vi "Inline HW RT Driver VI.vi"(7 "Operation":T1, 11 "Device Reference in":T2 format="%.0x") -> (0 "Error Code":i32)   [LabVIEW 2023, in "Waveform Analog Output Engine.lvlib"]
uses:
  Waveform Analog Output Engine.lvlib
  <vilib>/NI VeriStand/Custom Device API/Custom Device Item Ref.ctl
  <vilib>/NI VeriStand/Custom Device API/Hardware Interface Driver VI Operation.ctl
  <vilib>/NI VeriStand/Custom Device API/Custom Device Channel Type.ctl
  <vilib>/NI VeriStand/Custom Device API/Data Access Type.ctl
  <vilib>/NI VeriStand/Custom Device API/Block Data Reference.ctl
  <vilib>/NI VeriStand/Custom Device API/Data Reference.ctl
  DAQ Config Data.ctl
  Shared/Constants.vi
  <vilib>/NI VeriStand/Custom Device API/Global Data Refs.vi
  <vilib>/NI VeriStand/Custom Device API/Custom Device API.lvlib
  <resource>/objmgr/daqmx.rc
  Shared/Waveform Analog Output Shared.lvlib
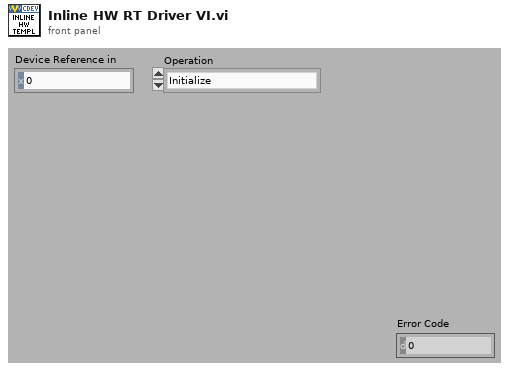
[diagram p1: front panel]
types:
  T1 = typedef "Custom Device API.lvlib/Hardware Interface Driver VI Operation.ctl" = enum16{"Initialize", "Start", "Read Data from HW", "Write Data to HW", "Close"}
  T2 = typedef "Custom Device API.lvlib/Custom Device Item Ref.ctl" = u64
  T3 = typedef "Custom Device API.lvlib/Block Data Reference.ctl" = cluster{"Data Reference":T4, "Offset":u64, "Length":u64}
  T4 = typedef "Custom Device API.lvlib/Data Reference.ctl" = i32
  T5 = typedef "Waveform Analog Output Engine.lvlib/DAQ Config Data.ctl" = cluster{"DAQ Physical Channel(s)":string, "SampleRate":dbl, "MaxV":dbl, "MinV":dbl, "#Samples":dbl, "StartDelay(ms)":dbl, "#OutputBuffers":dbl, "# Channels":i32, "Actual Sample Rate":dbl, "DAQ Ref Out":refnum<k21>, "Latency":dbl}
  T6 = cluster{"Input Data Refs":T3[], "Input Values Array":dbl[], "Output Data Refs":T3[], "Output Values Array":dbl[], "System Config Data":T5, "Error":errorcluster, "Waveform Parameter FIFO":refnum<k33>}
  T7 = cluster{"read mode":enum16{"polling", "blocking"}, "write mode":enum16{"polling", "blocking"}}
  T8 = cluster{"Hw Max":dbl, "Hw Min":dbl, "Requested Amplitude":dbl, "Requested Offset":dbl, "Coerced Amplitude":dbl, "Coerced Offset":dbl}
  T9 = typedef "Custom Device API.lvlib/Data Access Type.ctl" = enum16{"Read", "Write"}
  T10 = typedef "Custom Device API.lvlib/Custom Device Channel Type.ctl" = enum16{"Input", "Output"}
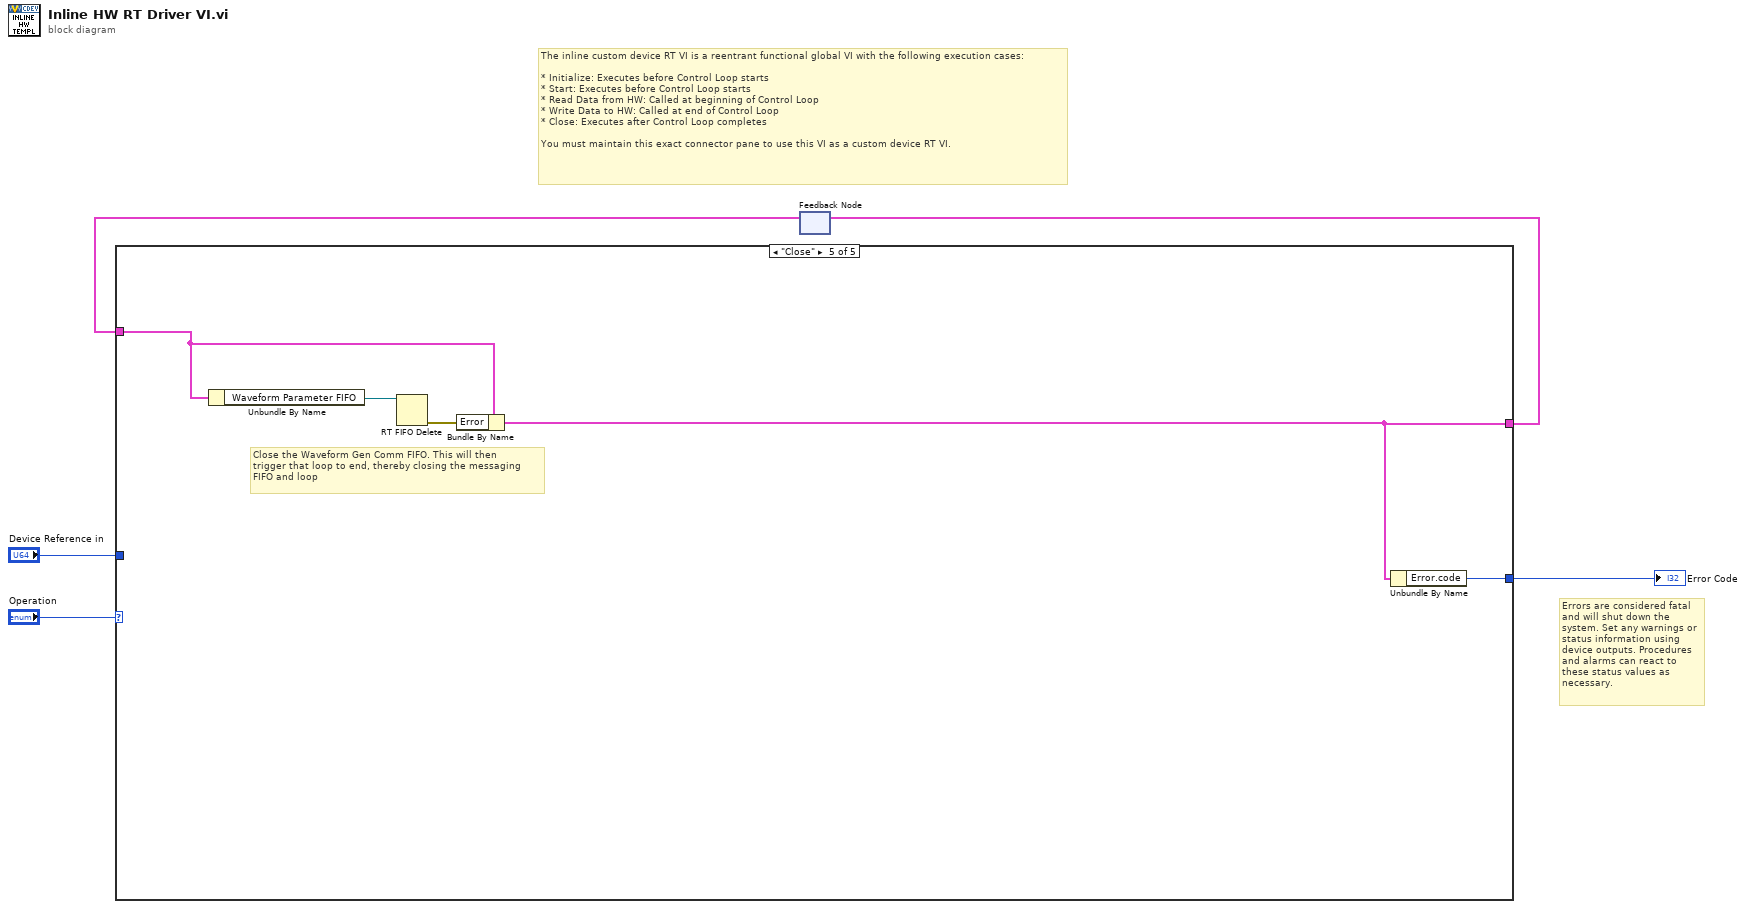
[diagram p0: block diagram]
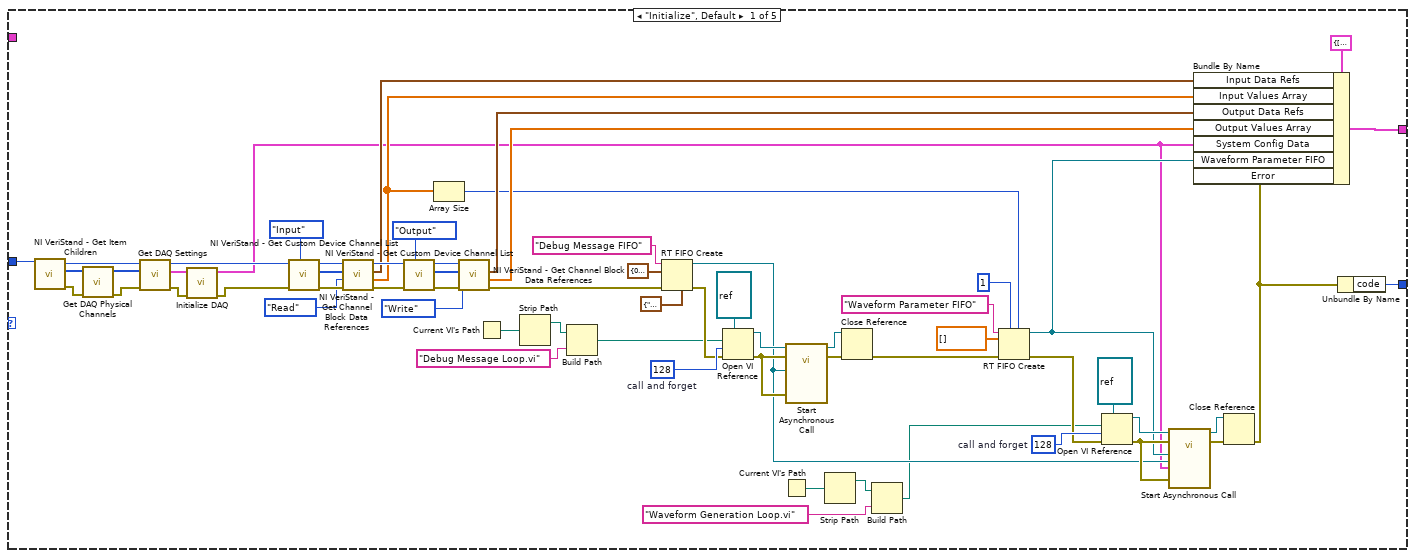
[diagram p2: hidden frame]
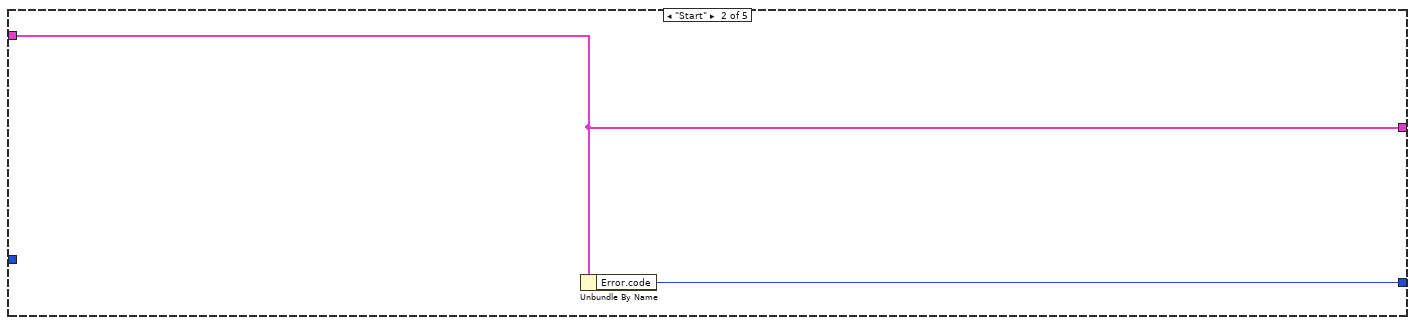
[diagram p3: hidden frame]
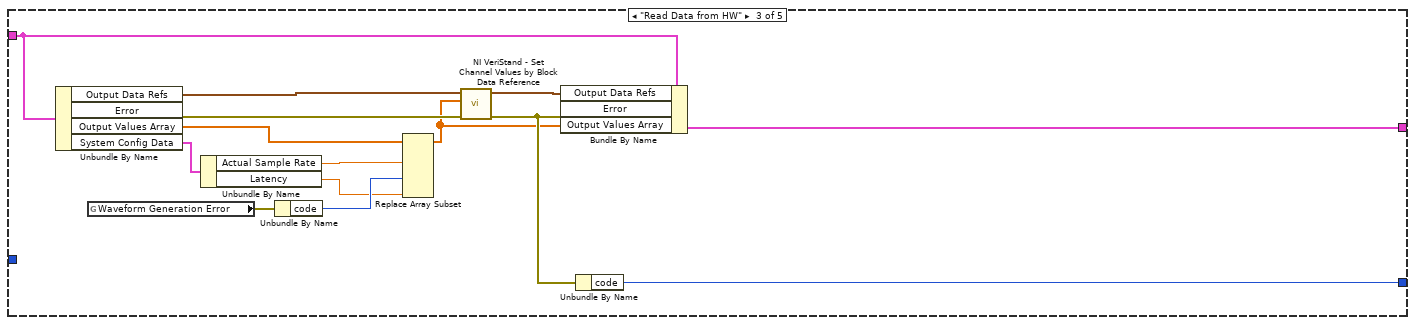
[diagram p4: hidden frame]
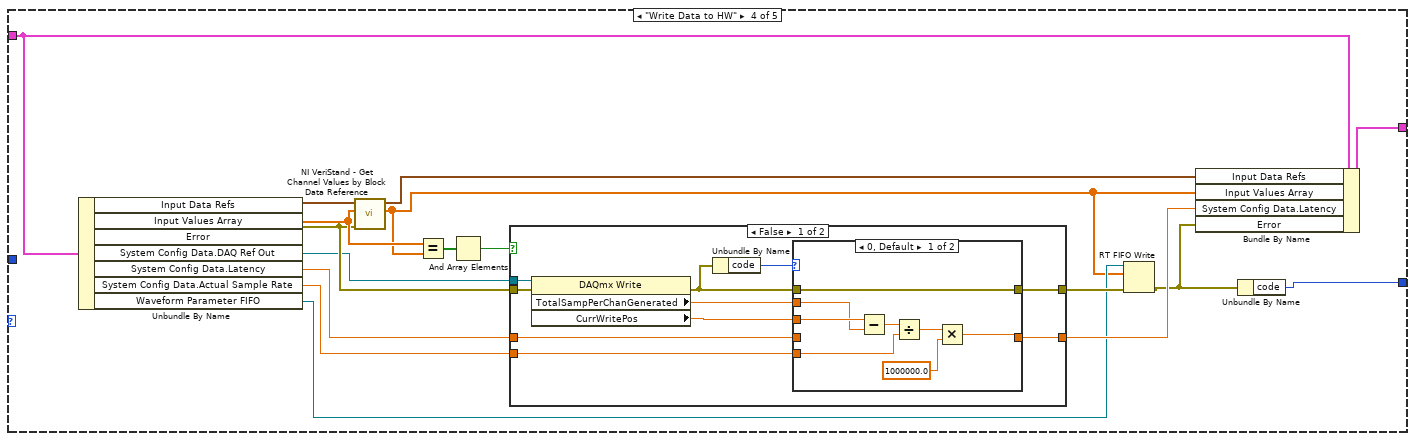
[diagram p5: hidden frame]
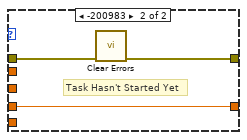
[diagram p6: hidden frame]
diagram:
  # "Errors are considered fatal and will shut down the system. Set any warnings or status information using device outputs. Procedures and alarms can react to these status values as necessary."
  # "The inline custom device RT VI is a reentrant functional global VI with the following execution cases:\n\n* Initialize: Executes before Control Loop starts\n* Start: Executes before Control Loop starts\n* Read Data from HW: Called at beginning of Control Loop\n* Write Data to HW: Called at end of Control Loop\n* Close: Executes after Control Loop completes\n\nYou must maintain this exact connector pane to use this VI as a custom device RT VI."
  n1 = feedback #1() -> (w3:T6)  [unwired: 1 out]
  n2 = case shown="\"Close\"" "Operation" {
    tunnel: [w45 w70 w83 w101 w126] -> w4
    tunnel: w3 -> [_ w70 w84 w102 w127]
    tunnel: "Device Reference in" -> [w60 _ _ _ _]
    tunnel: [w69 w71 w85 w100 w130] -> w1
    frame "Initialize", Default {
      w31 = 128  # call and forget
      w33 = 128  # call and forget
      n3 = call <vilib>:"NI VeriStand - Get Item Children.vi"("Item Ref in"=w60) -> ("error out"=w62:errorcluster, "Child Refs"=w61:T2[], "Item Ref out"=w66:T2)  [unwired: 7 in, 1 out]
      n4 = call "Get DAQ Physical Channels.vi"("error in (no error)"=w62, "DAQ Channel Section Refs"=w61) -> ("error out"=w67:errorcluster, "Physical Channels"=w65:i32[])  [unwired: 8 in]
      n5 = call "Get DAQ Settings.vi"("error in (no error)"=w67, "Physical Chan Array"=w65, "Device Ref in"=w66) -> ("error out"=w44:errorcluster, "DAQ Config Data"=w43:T5, "Device Ref Out"=w68:T2)  [unwired: 6 in]
      n6 = call "Initialize DAQ.vi"("error in (no error)"=w44, "DAQ Config Data In"=w43) -> ("error out"=w42:errorcluster, "DAQ Config Data Out"=w15:T5)  [unwired: 8 in]
      n7 = call <vilib>:"NI VeriStand - Get Custom Device Channel List.vi"("Channel Type"=Custom_Device_Channel_Type."Input", "error in (no error)"=w42, "Device Ref in"=w68) -> ("error out"=w58:errorcluster, "Specified Channel Ref List"=w57:T2[], "Device Ref out"=w59:T2)  [unwired: 6 in]
      n8 = call <vilib>:"NI VeriStand - Get Channel Block Data References.vi"("error in (no error)"=w58, "Access"=Data_Access_Type."Read", "Channel Refs"=w57, "Device Ref in"=w59) -> ("error out"=w54:errorcluster, "Values Array"=w21:dbl[], "Block Data Refs"=w48:T3[], "Device Ref out"=w55:T2)  [unwired: 4 in]
      n9 = call <vilib>:"NI VeriStand - Get Custom Device Channel List.vi"("Channel Type"=Custom_Device_Channel_Type."Output", "error in (no error)"=w54, "Device Ref in"=w55) -> ("error out"=w53:errorcluster, "Specified Channel Ref List"=w52:T2[], "Device Ref out"=w51:T2)  [unwired: 6 in]
      n10 = Array Size(array=w21) -> (size(s)=w20:i32)
      n11 = call <vilib>:"NI VeriStand - Get Channel Block Data References.vi"("error in (no error)"=w53, "Access"=Data_Access_Type."Write", "Channel Refs"=w52, "Device Ref in"=w51) -> ("error out"=w39:errorcluster, "Values Array"=w46:dbl[], "Block Data Refs"=w47:T3[])  [unwired: 4 in, 1 out]
      n12 = Current VI's Path() -> (path=w14:path)
      n13 = Strip Path(path=w14) -> (stripped path=w13:path)  [unwired: 1 out]
      n14 = Build Path(base path=w13, name or relative path="Debug Message Loop.vi" ("name (unnamed)")) -> (appended path=w11:path)
      n15 = RT FIFO Create(0:"Debug Message FIFO" ("name (unnamed)"), 1:T8 {"Hw Max"=0.0, "Hw Min"=0.0, "Requested Amplitude"=0.0, "Requested Offset"=0.0, "Coerced Amplitude"=0.0, "Coerced Offset"=0.0} ("Message Values"), 3:w39, 7:T7 {"read mode"=enum."blocking", "write mode"=enum."polling"} ("r/w modes (polling,polling)")) -> (8:w16:refnum<k33>, 11:w32:errorcluster)  [unwired: 4 in, 1 out]
      n16 = Open VI Reference(type specifier VI Refnum (for type only)=refnum<vi> refnum, vi path=w11, options=w33, error in (no error)=w32) -> (vi reference=w36:refnum<vi>, error out=w34:errorcluster)  [unwired: 2 in]
      n17 = Current VI's Path() -> (path=w9:path)
      n18 = call-by-ref "Start Asynchronous Call"(reference=w36, error in=w34, 8:"error in (no error)"=w34, "Refnum in"=w16) -> (reference out=w38:refnum<vi>, error out=w37:errorcluster)  [unwired: 9 in, 1 out]
      n19 = Strip Path(path=w9) -> (stripped path=w10:path)  [unwired: 1 out]
      n20 = Close Reference(reference=w38, error in (no error)=w37) -> (error out=w24:errorcluster)
      n21 = Build Path(base path=w10, name or relative path="Waveform Generation Loop.vi" ("name (unnamed)")) -> (appended path=w7:path)
      n22 = RT FIFO Create(0:"Waveform Parameter FIFO" ("name (unnamed)"), 1:dbl[] [], 3:w24, 4:u32 1 ("size (10)"), 6:w20) -> (8:w17:refnum<k33>, 11:w19:errorcluster)  [unwired: 3 in, 1 out]
      n23 = Open VI Reference(type specifier VI Refnum (for type only)=refnum<vi> refnum, vi path=w7, options=w31, error in (no error)=w19) -> (vi reference=w26:refnum<vi>, error out=w30:errorcluster)  [unwired: 2 in]
      n24 = call-by-ref "Start Asynchronous Call"(reference=w26, error in=w30, "Waveform Parameter FIFO"=w17, "Debugging RT FIFO"=w16, "DAQ Config Data Out"=w15, 11:"error in (no error)"=w30) -> (reference out=w27:refnum<vi>, error out=w28:errorcluster)  [unwired: 12 in]
      n25 = Close Reference(reference=w27, error in (no error)=w28) -> (error out=w18:errorcluster)
      n26 = Bundle By Name(cluster=T6 {"Input Data Refs"=[], "Input Values Array"=[], "Output Data Refs"=[], "Output Values Array"=[], "System Config Data"={"DAQ Physical Channel(s)"="", "SampleRate"=0.0, "MaxV"=0.0, "MinV"=0.0, "#Samples"=0.0, "StartDelay(ms)"=0.0, "#OutputBuffers"=0.0, "# Channels"=0, "Actual Sample Rate"=0.0, "DAQ Ref Out"="", "Latency"=0.0}, "Error"={"status"=FALSE, "code"=0, "source"=""}, "Waveform Parameter FIFO"=refnum}, "Input Data Refs"=w48, "Input Values Array"=w21, "Output Data Refs"=w47, "Output Values Array"=w46, "System Config Data"=w15, "Waveform Parameter FIFO"=w17, "Error"=w18) -> (w45:T6)
      n27 = Unbundle By Name(w18) -> ("code"=w69:i32)
    }
    frame "Start" {
      n28 = Unbundle By Name(w70) -> ("Error.code"=w71:i32)
    }
    frame "Read Data from HW" {
      n29 = Unbundle By Name(w84) -> ("Output Data Refs"=w82:T3[], "Error"=w79:errorcluster, "Output Values Array"=w81:dbl[], "System Config Data"=w80:T5)
      n30 = global read "Constants.vi" "Waveform Generation Error"() -> (w72:errorcluster)
      n31 = Unbundle By Name(w80) -> ("Actual Sample Rate"=w77:dbl, "Latency"=w76:dbl)
      n32 = Unbundle By Name(w72) -> ("code"=w78:i32)
      n33 = Replace Array Subset(array=w81, new element #1=w77, new element #2=w78, new element #3=w76) -> (w73:dbl[])  [unwired: 3 in]
      n34 = call <vilib>:"NI VeriStand - Set Channel Values by Block Data Reference.vi"("error in (no error)"=w79, "Values Array in"=w73, "Block Data Ref"=w82) -> ("error out"=w74:errorcluster, "Block Data Ref dup"=w75:T3[])  [unwired: 6 in, 1 out]
      n35 = Bundle By Name(cluster=w84, "Output Data Refs"=w75, "Error"=w74, "Output Values Array"=w73) -> (w83:T6)
      n36 = Unbundle By Name(w74) -> ("code"=w85:i32)
    }
    frame "Write Data to HW" {
      n37 = Unbundle By Name(w102) -> ("Input Data Refs"=w99:T3[], "Input Values Array"=w96:dbl[], "Error"=w94:errorcluster, "System Config Data.DAQ Ref Out"=w90:refnum<k21>, "System Config Data.Latency"=w93:dbl, "System Config Data.Actual Sample Rate"=w91:dbl, "Waveform Parameter FIFO"=w88:refnum<k33>)
      n38 = call <vilib>:"NI VeriStand - Get Channel Values by Block Data Reference.vi"("error in (no error)"=w94, "Values Array in"=w96, "Block Data Ref"=w99) -> ("Values Array out"=w86:dbl[], "Block Data Ref dup"=w95:T3[])  [unwired: 6 in, 1 out]
      n39 = Equal?(x=w96, y=w86) -> (x = y?=w97:bool[])
      n40 = And Array Elements(Boolean array=w97) -> (logical AND=w98:bool)
      n41 = case shown="False" w98 {
        tunnel: w90 -> [w107 _]
        tunnel: w94 -> [w112 w125]
        tunnel: [w103 w125] -> w89
        tunnel: w93 -> [w104 w124]
        tunnel: [w108 w124] -> w92
        tunnel: w91 -> [w109 _]
        frame False {
          n42 = property class="DAQmx Write"(reference=w107, error in=w112) -> (error out=w105:errorcluster, "TotalSampPerChanGenerated"=w110:dbl, "CurrWritePos"=w111:dbl)  [unwired: 1 out]
          n43 = Unbundle By Name(w105) -> ("code"=w106:i32)
          n44 = case shown="0, Default" w106 {
            tunnel: w111 -> [w120 _]
            tunnel: w110 -> [w119 _]
            tunnel: w109 -> [w117 _]
            tunnel: [w113 w123] -> w108
            tunnel: w105 -> [w114 w122]
            tunnel: w104 -> [_ w123]
            tunnel: [w114 w121] -> w103
            frame 0, Default {
              n45 = Subtract(x=w120, y=w119) -> (x-y=w118:dbl)
              n46 = Divide(x=w118, y=w117) -> (x/y=w116:dbl)
              n47 = Multiply(x=w116, y=1000000.0) -> (x*y=w113:dbl)
            }
            frame -200983 {
              # "Task Hasn't Started Yet"
              n48 = call <vilib>:"Clear Errors.vi"("error in (no error)"=w122) -> ("error out"=w121:errorcluster)  [unwired: 5 in, 1 out]
            }
          }
        }
        frame True {
        }
      }
      n49 = RT FIFO Write(0:w88, 1:w86, 3:w89) -> (11:w87:errorcluster)  [unwired: 2 in, 3 out]
      n50 = Bundle By Name(cluster=w102, "Input Data Refs"=w95, "Input Values Array"=w86, "System Config Data.Latency"=w92, "Error"=w87) -> (w101:T6)
      n51 = Unbundle By Name(w87) -> ("code"=w100:i32)
    }
    frame "Close" {
      # "Close the Waveform Gen Comm FIFO. This will then\ntrigger that loop to end, thereby closing the messaging\nFIFO and loop"
      n52 = Unbundle By Name(w127) -> ("Waveform Parameter FIFO"=w129:refnum<k33>)
      n53 = RT FIFO Delete(0:w129) -> (11:w128:errorcluster)  [unwired: 2 in]
      n54 = Bundle By Name(cluster=w127, "Error"=w128) -> (w126:T6)
      n55 = Unbundle By Name(w126) -> ("Error.code"=w130:i32)
    }
  }
  "Error Code" <- w1
  n56 = feedback-in #1(w4) -> ()
